vi "Update Header.vi"(8 "error in (no error)":errorcluster, 11 "CIFFIFO in":refnum<class "CIFfifo.lvclass">) -> (0 "error out":errorcluster, 3 "CIFFIFO out":refnum<class "CIFfifo.lvclass">)   [LabVIEW 2021, in "CIFfifo.lvclass"]
uses:
  CIFfifo.lvclass
  CIFfifo.lvclass/CIFfifo.ctl
  ChannelCommon.lvlib
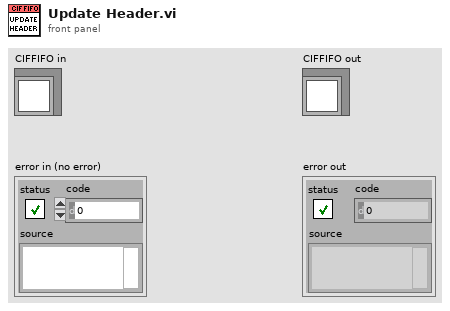
[diagram p1: front panel]
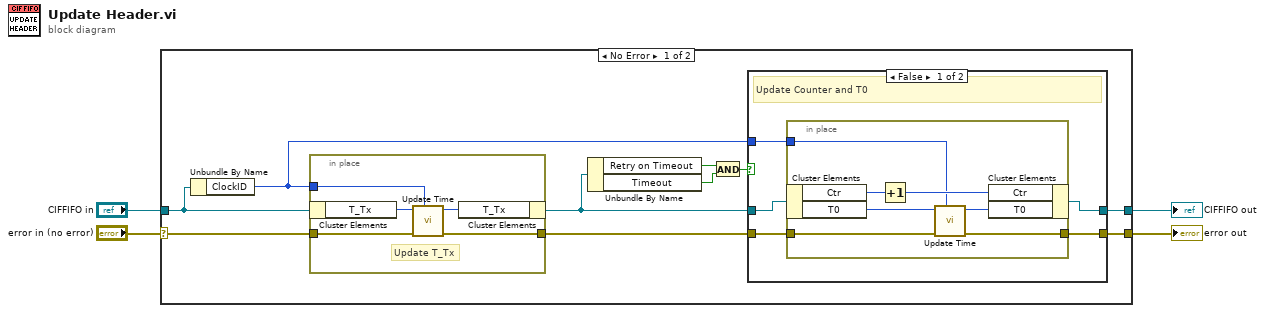
[diagram p0: block diagram]
diagram:
  n1 = case shown="No Error" "error in (no error)" {
    selector: "error in (no error)" -> [w11 w35]
    tunnel: [w8 w35] -> w3
    tunnel: [w7 w34] -> w1
    tunnel: "CIFFIFO in" -> [w6 w34]
    frame No Error {
      n2 = Unbundle By Name(w6) -> ("ClockID"=w5:u8)
      n3 = in-place {
        in-place-border: w11 -> [w17]
        in-place-border: [w16] -> w10
        in-place-border: w5 -> [w15]
        # "Update T_Tx"
        n4 = in-place-cluster #1(w6) -> ("T_Tx"=w19:u64)
        n5 = call "Update Time.vi"("ClockID"=w15, "error in (no error)"=w17, "Time in"=w19) -> ("error out"=w16:errorcluster, "Time out"=w18:u64)  [unwired: 7 in]
        n6 = in-place-cluster #1("T_Tx"=w18) -> (w9:refnum<class "CIFfifo.lvclass">)
      }
      n7 = Unbundle By Name(w9) -> ("Retry on Timeout"=w14:bool, "Timeout"=w13:bool)
      n8 = And(x=w14, y=w13) -> (x .and. y?=w12:bool)
      n9 = case shown="False" w12 {
        tunnel: w9 -> [w24 w33]
        tunnel: [w22 w33] -> w7
        tunnel: w10 -> [w23 w32]
        tunnel: [w21 w32] -> w8
        tunnel: w5 -> [w20 _]
        frame False {
          # "Update Counter and T0"
          n10 = in-place {
            in-place-border: w23 -> [w27]
            in-place-border: [w26] -> w21
            in-place-border: w20 -> [w25]
            n11 = in-place-cluster #2(w24) -> ("Ctr"=w31:u64, "T0"=w29:u64)
            n12 = Increment(x=w31) -> (x+1=w30:u64)
            n13 = call "Update Time.vi"("ClockID"=w25, "error in (no error)"=w27, "Time in"=w29) -> ("error out"=w26:errorcluster, "Time out"=w28:u64)  [unwired: 7 in]
            n14 = in-place-cluster #2("Ctr"=w30, "T0"=w28) -> (w22:refnum<class "CIFfifo.lvclass">)
          }
        }
        frame True {
          # "Retry last packet"
        }
      }
    }
    frame Error {
    }
  }
  "error out" <- w3
  "CIFFIFO out" <- w1
